vi "Move_Trav_and_Meas.vi"() -> ()   [LabVIEW 2011]
uses:
  Controls/Post_Process.ctl
  Controls/User_Specific_mode.ctl
  Gen Trav/Trav_mode.ctl
  Controls/Positions.ctl
  Globals/Meas_global.vi
  Globals/Trav_pos_global.vi
  Globals/Dynamic_call_global.ph.vi
panel:
  out "Current Trav Position":dbl[](array[numeric])
  in  "Traverse Speed Factor":dbl=1.0
  in  "Traverse Name (leave blank for default)":string
  out "Plug in titles":string[](array[string])
  out "Plug in values":string[](array[string])
  in  "Position":dbl[](array[numeric])=[0.0, 0.0, 0.0]
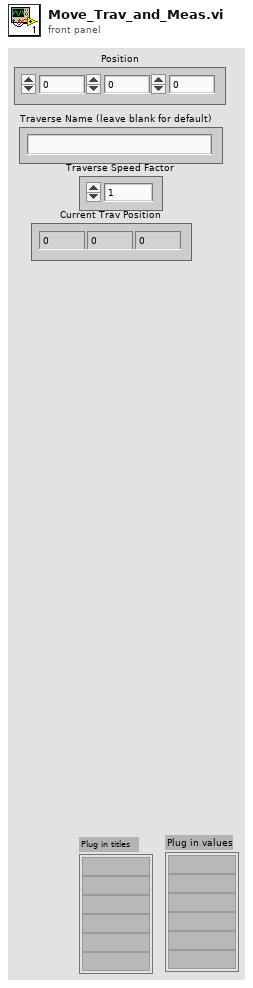
[diagram p1: front panel]
types:
  T1 = typedef "Post_Process.ctl" = enum16{"Take New Data", "Post Process Raw Data File"}
  T2 = typedef "User_Specific_mode.ctl" = enum16{"Check VI only", "Run VI"}
  T3 = typedef "Trav_mode.ctl" = enum16{"Move traverse", "Read traverse position", "Teach Position"}
  T4 = typedef "Positions.ctl" = enum16{"X", "Y", "Z", "XY", "XZ", "YZ", "XYZ"}
  T5 = typedef "Rendezvous RefNum" = refnum<k1>
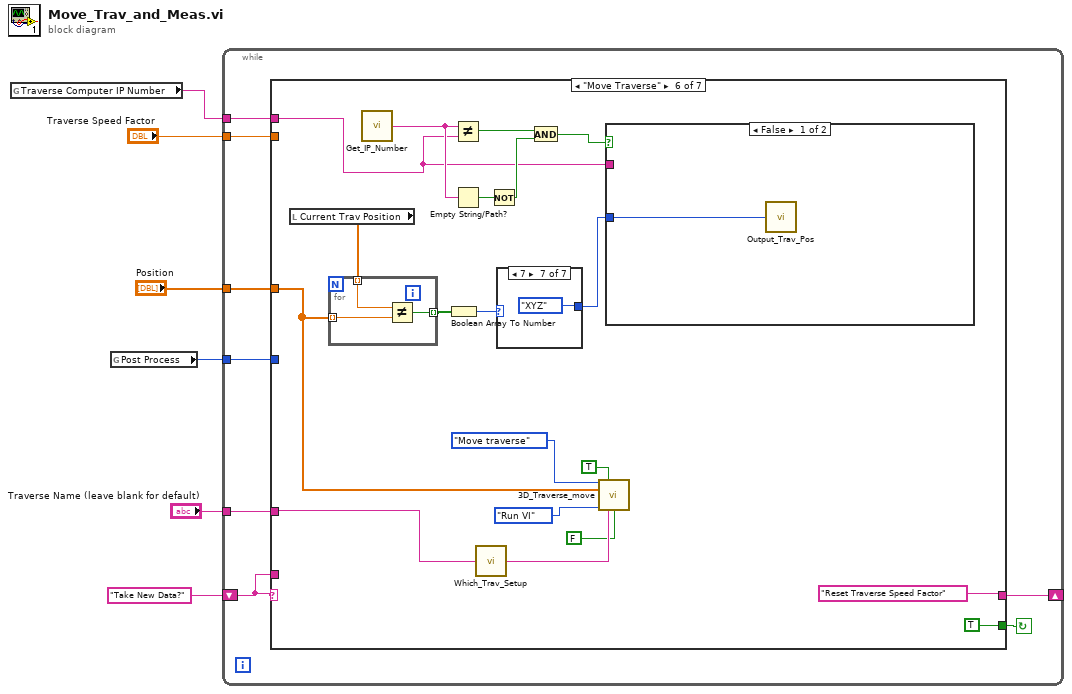
[diagram p0: block diagram]
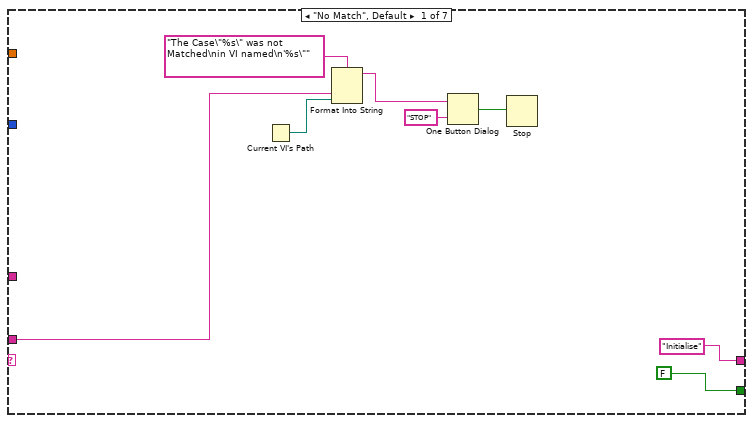
[diagram p2: hidden frame]
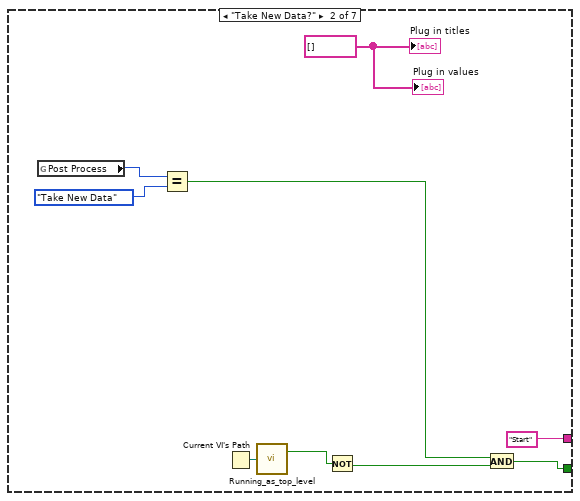
[diagram p3: hidden frame]
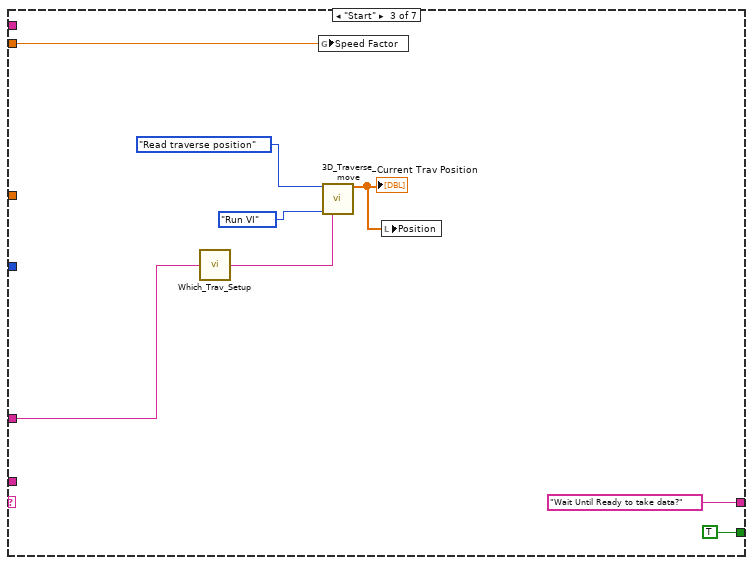
[diagram p4: hidden frame]
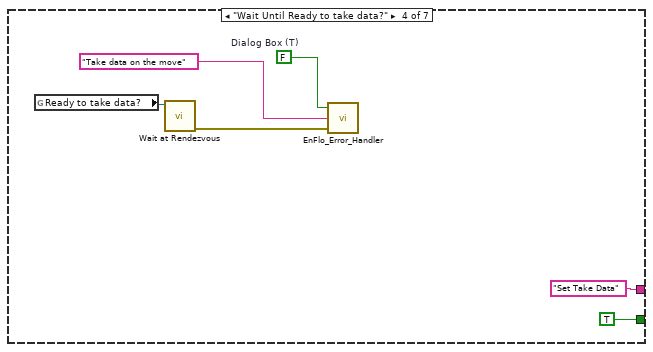
[diagram p5: hidden frame]
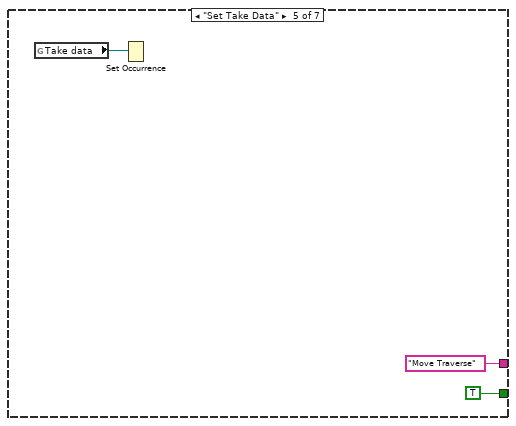
[diagram p6: hidden frame]
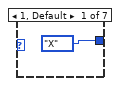
[diagram p7: hidden frame]
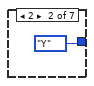
[diagram p8: hidden frame]
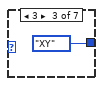
[diagram p9: hidden frame]
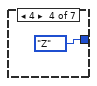
[diagram p10: hidden frame]
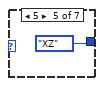
[diagram p11: hidden frame]
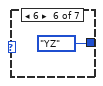
[diagram p12: hidden frame]
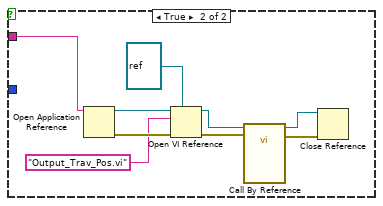
[diagram p13: hidden frame]
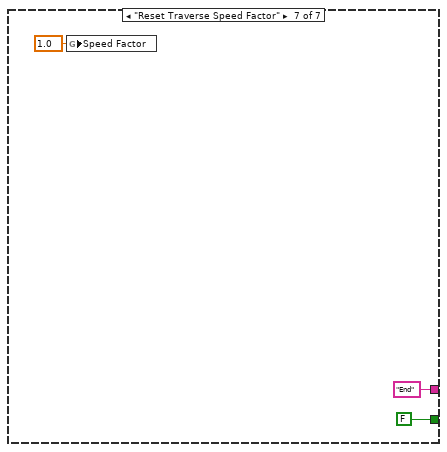
[diagram p14: hidden frame]
diagram:
  n1 = global read "Trav_pos_global.vi" "Traverse Computer IP Number"() -> (w1:string)
  n2 = global read "Meas_global.vi" "Post Process"() -> (w5:T1)
  n3 = while {
    shift-left: "Take New Data?" -> [w12]
    shift-right: [w13] -> _
    tunnel: w5 -> [w11]
    tunnel: "Position" -> [w10]
    tunnel: "Traverse Name (leave blank for default)" -> [w9]
    tunnel: "Traverse Speed Factor" -> [w8]
    tunnel: w1 -> [w7]
    stop <- w14 continue-if-true
    n4 = case shown="\"Move Traverse\"" w12 {
      tunnel: [FALSE w25 TRUE ("Command Found") TRUE ("Command Found") TRUE ("Command Found") TRUE ("Command Found") FALSE ("Command Found")] -> w14
      tunnel: ["Initialise" "Start" "Wait Until Ready to take data?" ("f") "Set Take Data" "Move Traverse" "Reset Traverse Speed Factor" "End" ("f")] -> w13
      tunnel: w12 -> [w17 _ _ _ _ _ _]
      tunnel: w11 -> [_ _ _ _ _ _ _]
      tunnel: w10 -> [_ _ _ _ _ w53 _]
      tunnel: w9 -> [_ _ w33 _ _ w60 _]
      tunnel: w8 -> [_ _ w38 _ _ _ _]
      tunnel: w7 -> [_ _ _ _ _ w54 _]
      frame "No Match", Default {
        n5 = Current VI's Path() -> (path=w16:path)
        n6 = Format Into String(format string="The Case\"%s\" was not Matched\nin VI named\n'%s\"" ("Format String"), w17, w16) -> (resulting string=w20:string)  [unwired: 2 in, 1 out]
        n7 = One Button Dialog(message=w20, button name ("OK")="STOP") -> (true=w18:bool)
        n8 = Stop(stop? (T)=w18) -> ()
      }
      frame "Take New Data?" {
        w28 = string[] [] ("Plug in titles")
        n9 = global read "Meas_global.vi" "Post Process"() -> (w30:T1)
        n10 = Equal?(x=w30, y=Post_Process."Take New Data" ("Post Process")) -> (x = y?=w26:bool)
        n11 = Current VI's Path() -> (path=w27:path)
        n12 = call "Running_as_top_level.vi"("Vi path name"=w27) -> ("Top Level"=w24:bool)  [unwired: 1 out]
        n13 = Not(x=w24) -> (.not. x?=w23:bool)
        n14 = And(x=w26, y=w23) -> (x .and. y?=w25:bool)
        "Plug in titles" <- w28
        "Plug in values" <- w28
      }
      frame "Start" {
        n15 = call "Which_Trav_Setup.vi"("Extra Command String"=w33) -> ("Traverse Setup"=w34:string)
        n16 = global write "Trav_pos_global.vi" "Speed Factor"(w38) -> ()
        n17 = call "3D_Traverse_move.vi"("Mode"=Trav_mode."Read traverse position", "Simulate/Run"=User_Specific_mode."Run VI", "Traverse name"=w34) -> ("Trav Position achieved"=w32:dbl[])  [unwired: 10 in, 2 out]
        "Current Trav Position" <- w32
        n18 = local write "Position"(w32) -> ()
      }
      frame "Wait Until Ready to take data?" {
        w41 = FALSE  # Dialog Box (T)
        n19 = global read "Dynamic_call_global.ph.vi" "Ready to take data?"() -> (w44:T5)
        n20 = call <vilib>:"Wait at Rendezvous.vi"("rendezvous"=w44) -> ("error out"=w42:errorcluster)  [unwired: 4 in, 2 out]
        n21 = call "EnFlo_Error_Handler.vi"("error in (no error)"=w42, "Error Type"="Take data on the move", "Dialog Box (T)"=w41) -> ()  [unwired: 3 out]
      }
      frame "Set Take Data" {
        n22 = global read "Dynamic_call_global.ph.vi" "Take data"() -> (w46:refnum<k4>)
        n23 = Set Occurrence(w46) -> ()
      }
      frame "Move Traverse" {
        n24 = local read "Current Trav Position"() -> (w52:dbl[])
        n25 = for {
          tunnel: w53 -> [w77] mode=indexing
          tunnel: w52 -> [w76] mode=indexing
          tunnel: [w75] -> w51 mode=indexing
          n26 = Not Equal?(x=w76, y=w77) -> (x != y?=w75:bool)
        }
        n27 = call "Get_IP_Number.vi"() -> ("IP Number"=w55:string)
        n28 = Boolean Array To Number(Boolean array=w51) -> (number=w50:u32)
        n29 = Not Equal?(x=w55, y=w54) -> (x != y?=w57:bool)
        n30 = Empty String/Path?(string/path=w55) -> (empty?=w59:bool)
        n31 = call "Which_Trav_Setup.vi"("Extra Command String"=w60) -> ("Traverse Setup"=w63:string)
        n32 = Not(x=w59) -> (.not. x?=w58:bool)
        n33 = case shown="7" w50 {
          tunnel: [Positions."X" ("Positions to Output") Positions."Y" ("Positions to Output") Positions."XY" ("Positions to Output") Positions."Z" ("Positions to Output") Positions."XZ" ("Positions to Output") Positions."YZ" ("Positions to Output") Positions."XYZ" ("Positions to Output")] -> w49
          frame 1, Default {
          }
          frame 2 {
          }
          frame 3 {
          }
          frame 4 {
          }
          frame 5 {
          }
          frame 6 {
          }
          frame 7 {
          }
        }
        n34 = And(x=w57, y=w58) -> (x .and. y?=w56:bool)
        n35 = call "3D_Traverse_move.vi"("Mode"=Trav_mode."Move traverse", "Route Checking?"=TRUE, "Position"=w53, "Simulate/Run"=User_Specific_mode."Run VI", "Traverse name"=w63, "Backlash Compensation?"=FALSE) -> ()  [unwired: 7 in, 3 out]
        n36 = case shown="False" w56 {
          tunnel: w54 -> [_ w83]
          tunnel: w49 -> [w78 _]
          frame False {
            n37 = call "Output_Trav_Pos.vi"("Positions to Output"=w78) -> ()  [unwired: 4 in, 1 out]
          }
          frame True {
            n38 = Open Application Reference(11:w83) -> (0:w87:errorcluster, 3:w81:refnum<vi>)  [unwired: 2 in, 1 out]
            n39 = Open VI Reference(type specifier VI Refnum (for type only)=refnum<vi> refnum, application reference (local)=w81, vi path="Output_Trav_Pos.vi", error in (no error)=w87) -> (vi reference=w80:refnum<vi>, error out=w84:errorcluster)  [unwired: 2 out]
            n40 = call-by-ref "?"(reference=w80, error in=w84) -> (reference out=w86:refnum<vi>, error out=w85:errorcluster)  [unwired: 5 in, 1 out]
            n41 = Close Reference(reference=w86, error in (no error)=w85) -> ()  [unwired: 1 out]
          }
        }
      }
      frame "Reset Traverse Speed Factor" {
        n42 = global write "Trav_pos_global.vi" "Speed Factor"(1.0 ("Speed Factor")) -> ()
      }
    }
  }
